vi "LoopselFF_2cam.VI"() -> ()   [LabVIEW 2017]
panel:
  in  "nob slide":u32(slide)=27666 scale=1.0..6.0
  in  "no.of blocks (nob)":u32=6
  out "cams recognised":u8
  in  "cam select\n1: cam 1\n2: cam 2\n3: both cams":u8=3
  out "Signalverlaufgraph 2":u16[](graph)=[0, 0, 0, 0, 0, 1, 0, 27665, 0, 0, 0, 0, 0, 0, 0, 0, 0, 0, 0, 0, 0, 0, 0, 0, 0, 0, 0, 0, 0, 0, 0, 0, 0, 0, 0, 0, 0, 0, 0, 0, 0, 0, 0, 0, 0, 0, 0, 0, 0, 0, 0, 0, 0, 0, 0, 0, 0, 0, 0, 0, 0, 0, 0, 0, 0, 0, 0, 0, 0, 0, 0, 0, 0, 0, 0, 0, 0, 0, 0, 0, 0, 0, 0, 0, 0, 0, 0, 0, 0, 0, 0, 0, 0, 0, 0, 0, 0, 0, 0, 0, 0, 0, 0, 0, 0, 0, 0, 0, 0, 0, 0, 0, 0, 0, 0, 0, 0, 0, 0, 0, 0, 0, 0, 0, 0, 0, 0, 0, 0, 0, 0, 0, 0, 0, 0, 0, 0, 0, 0, 0, 0, 0, 0, 0, 0, 0, 0, 0, 0, 0, 0, 0, 0, 0, 0, 0, 0, 0, 0, 0, 0, 0, 0, 0, 0, 0, 0, 0, 0, 0, 0, 0, 0, 0, 0, 0, 0, 0, 0, 0, 0, 0, 0, 0, 0, 0, 0, 0, 0, 0, 0, 0, 0, 0, 0, 0, 0, 0, 0, 0, 0, 0, 0, 0, 0, 0, 0, 0, 0, 0, 0, 0, 0, 0, 0, 0, 0, 0, 0, 0, 0, 0, 0, 0, 0, 0, 0, 0, 0, 0, 0, 0, 0, 0, 0, 0, 0, 0, 0, 0, 0, 0, 0, 0, 0, 0, 0, 0, 0, 0, 0, 0, 0, 0, 0, 0, 0, 0, 0, 0, 0, 0, 0, 0, 0, 0, 0, 0, 0, 0, 0, 0, 0, 0, 0, 0, 0, 0, 0, 0, 0, 0, 0, 0, 0, 0, 0, 0, 0, 0, 0, 0, 0, 0, 0, 0, 0, 0, 0, 0, 0, 0, 0, 0, 0, 0, 0, 0, 0, 0, 0, 0, 0, 0, 0, 0, 0, 0, 0, 0, 0, 0, 0, 0, 0, 0, 0, 0, 0, 0, 0, 0, 0, 0, 0, 0, 0, 0, 0, 0, 0, 0, 0, 0, 0, 0, 0, 0, 0, 0, 0, 0, 0, 0, 0, 0, 0, 0, 0, 0, 0, 0, 0, 0, 0, 0, 0, 0, 0, 0, 0, 0, 0, 0, 0, 0, 0, 0, 0, 0, 0, 0, 0, 0, 0, 0, 0, 0, 0, 0, 0, 0, 0, 0, 0, 0, 0, 0, 0, 0, 0, 0, 0, 0, 0, 0, 0, 0, 0, 0, 0, 0, 0, 0, 0, 0, 0, 0, 0, 0, 0, 0, 0, 0, 0, 0, 0, 0, 0, 0, 0, 0, 0, 0, 0, 0, 0, 0, 0, 0, 0, 0, 0, 0, 0, 0, 0, 0, 0, 0, 0, 0, 0, 0, 0, 0, 0, 0, 0, 0, 0, 0, 0, 0, 0, 0, 0, 0, 0, 0, 0, 0, 0, 0, 0, 0, 0, 0, 0, 0, 0, 0, 0, 0, 0, 0, 0, 0, 0, 0, 0, 0, 0, 0, 0, 0, 0, 0, 0, 0, 0, 0, 0, 0, 0, 0, 0, 0, 0, 0, 0, 0, 0, 0, 0, 0, 0, 0, 0, 0, 0, 0, 0, 0, 0, 0, 0, 0, 0, 0, 0, 0, 0, 0, 0, 0, 0, 0, 0, 0, 0, 0, 0, 0, 0, 0, 0, 0, 0, 0, 0, 0, 0, 0, 0, 0, 0, 0, 0, 0, 0, 0, 0, 0, 0, 0, 0, 0, 0, 0, 0, 0, 0, 0, 0, 0, 0, 0, 0, 0, 0, 0, 0, 0, 0, 0, 0, 0, 0, 0, 0, 0, 0, 0, 0, 0, 0, 0, 0, 0, 0, 0, 0, 0, 0, 0, 0, 0, 0, 0, 0, 0, 0, 0, 0, 0, 0, 0, 0, 0, 0, 0, 0, 0, 0, 0, 0, 0, 0, 0, 0, 0, 0, 0, 0, 0, 0, 0, 0, 0, 0, 0, 0, 0, 0, 0, 0, 0, 0, 0, 0, 0, 0, 0, 0, 0, 0, 0, 0, 0, 0, 0, 0, 0, 0, 0, 0, 0, 0, 0, 0, 0, 0, 0, 0, 0, 0, 0, 0, 0, 0, 0, 0, 0, 0, 0, 0, 0, 0, 0, 0, 0, 0, 0, 0, 0, 0, 0, 0, 0, 0, 0, 0, 0, 0, 0, 0, 0, 0, 0, 0, 0, 0, 0, 0, 0, 0, 0, 0, 0, 0, 0, 0, 0, 0, 0, 0, 0, 0, 0, 0, 0, 0, 0, 0, 0, 0, 0, 0, 0, 0, 0, 0, 0, 0, 0, 0, 0, 0, 0, 0, 0, 0, 0, 0, 0, 0, 0, 0, 0, 0, 0, 0, 0, 0, 0, 0, 0, 0, 0, 0, 0, 0, 0, 0, 0, 0, 0, 0, 0, 0, 0, 0, 0, 0, 0, 0, 0, 0, 0, 0, 0, 0, 0, 0, 0, 0, 0, 0, 0, 0, 0, 0, 0, 0, 0, 0, 0, 0, 0, 0, 0, 0, 0, 0, 0, 0, 0, 0, 0, 0, 0, 0, 0, 0, 0, 0, 0, 0, 0, 0, 0, 0, 0, 0, 0, 0, 0, 0, 0, 0, 0, 0, 0, 0, 0, 0, 0, 0, 0, 0, 0, 0, 0, 0, 0, 0, 0, 0, 0, 0, 0, 0, 0, 0, 0, 0, 0, 0, 0, 0, 0, 0, 0, 0, 0, 0, 0, 0, 0, 0, 0, 0, 0, 0, 0, 0, 0, 0, 0, 0, 0, 0, 0, 0, 0, 0, 0, 0, 0, 0, 0, 0, 0, 0, 0, 0, 0, 0, 0, 0, 0, 0, 0, 0, 0, 0, 0, 0, 0, 0, 0, 0, 0, 0, 0, 0, 0, 0, 0, 0, 0, 0, 0, 0, 0, 0, 0, 0, 0, 0, 0, 0, 0, 0, 0, 0, 0, 0, 0, 0, 0, 0, 0, 0, 0, 0, 0, 0, 0, 0, 0, 0, 0, 0, 0, 0, 0, 0, 0, 0, 0, 0, 0, 0, 0, 0, 0, 0, 0, 0, 0, 0, 0, 0, 0, 0, 0, 0, 0, 0, 0, 0, 0, 0, 0, 0, 0, 0, 0, 0, 0, 0, 0, 0, 0, 0, 0, 0, 0, 0, 0, 0, 0, 0, 0, 0, 0, 0, 0, 0, 0, 0, 0, 0, 0, 0, 0, 0, 0, 0, 0, 0, 0, 0, 0, 0, 0, 0, 0, 0, 0, 0, 0, 0, 0, 0, 0, 0, 0, 0, 0, 0, 0, 0, 0, 0, 0, 0, 0, 0, 0, 0, 0, 0, 0, 0, 0, 0, 0, 0, 0, 0, 0, 0, 0, 0, 0, 0, 0, 0, 0, 0, 0, 0, 0, 0, 0]
  in  "alloc mem":bool
  out "FREE \nRAM MB":u64=14179
  out "BUILT-IN\nRAM MB":u64=16662
  out "SEC":dbl=1.2
  out "MB RAM":u64=125
  in  "pos slope":u8=1
  in  "both slopes":u8
  in  "DAT in 10ns":u32
  in  "extTrig 0/1":u8
  in  "stop all":bool
  in  "start new block":bool
  in  "nos slide":u32(slide)=27666 scale=1.0..70000.0
  in  "frequency[Hz]":u32
  in  "no.of samples (nos)":u32=10000
  in  "exposuretime[ms]":dbl=0.02 format="%.3f"
  out "Signalverlaufgraph":u16[](graph)=[0, 0, 0, 0, 0, 1, 0, 27665, 0, 0, 0, 0, 0, 0, 0, 0, 0, 0, 0, 0, 0, 0, 0, 0, 0, 0, 0, 0, 0, 0, 0, 0, 0, 0, 0, 0, 0, 0, 0, 0, 0, 0, 0, 0, 0, 0, 0, 0, 0, 0, 0, 0, 0, 0, 0, 0, 0, 0, 0, 0, 0, 0, 0, 0, 0, 0, 0, 0, 0, 0, 0, 0, 0, 0, 0, 0, 0, 0, 0, 0, 0, 0, 0, 0, 0, 0, 0, 0, 0, 0, 0, 0, 0, 0, 0, 0, 0, 0, 0, 0, 0, 0, 0, 0, 0, 0, 0, 0, 0, 0, 0, 0, 0, 0, 0, 0, 0, 0, 0, 0, 0, 0, 0, 0, 0, 0, 0, 0, 0, 0, 0, 0, 0, 0, 0, 0, 0, 0, 0, 0, 0, 0, 0, 0, 0, 0, 0, 0, 0, 0, 0, 0, 0, 0, 0, 0, 0, 0, 0, 0, 0, 0, 0, 0, 0, 0, 0, 0, 0, 0, 0, 0, 0, 0, 0, 0, 0, 0, 0, 0, 0, 0, 0, 0, 0, 0, 0, 0, 0, 0, 0, 0, 0, 0, 0, 0, 0, 0, 0, 0, 0, 0, 0, 0, 0, 0, 0, 0, 0, 0, 0, 0, 0, 0, 0, 0, 0, 0, 0, 0, 0, 0, 0, 0, 0, 0, 0, 0, 0, 0, 0, 0, 0, 0, 0, 0, 0, 0, 0, 0, 0, 0, 0, 0, 0, 0, 0, 0, 0, 0, 0, 0, 0, 0, 0, 0, 0, 0, 0, 0, 0, 0, 0, 0, 0, 0, 0, 0, 0, 0, 0, 0, 0, 0, 0, 0, 0, 0, 0, 0, 0, 0, 0, 0, 0, 0, 0, 0, 0, 0, 0, 0, 0, 0, 0, 0, 0, 0, 0, 0, 0, 0, 0, 0, 0, 0, 0, 0, 0, 0, 0, 0, 0, 0, 0, 0, 0, 0, 0, 0, 0, 0, 0, 0, 0, 0, 0, 0, 0, 0, 0, 0, 0, 0, 0, 0, 0, 0, 0, 0, 0, 0, 0, 0, 0, 0, 0, 0, 0, 0, 0, 0, 0, 0, 0, 0, 0, 0, 0, 0, 0, 0, 0, 0, 0, 0, 0, 0, 0, 0, 0, 0, 0, 0, 0, 0, 0, 0, 0, 0, 0, 0, 0, 0, 0, 0, 0, 0, 0, 0, 0, 0, 0, 0, 0, 0, 0, 0, 0, 0, 0, 0, 0, 0, 0, 0, 0, 0, 0, 0, 0, 0, 0, 0, 0, 0, 0, 0, 0, 0, 0, 0, 0, 0, 0, 0, 0, 0, 0, 0, 0, 0, 0, 0, 0, 0, 0, 0, 0, 0, 0, 0, 0, 0, 0, 0, 0, 0, 0, 0, 0, 0, 0, 0, 0, 0, 0, 0, 0, 0, 0, 0, 0, 0, 0, 0, 0, 0, 0, 0, 0, 0, 0, 0, 0, 0, 0, 0, 0, 0, 0, 0, 0, 0, 0, 0, 0, 0, 0, 0, 0, 0, 0, 0, 0, 0, 0, 0, 0, 0, 0, 0, 0, 0, 0, 0, 0, 0, 0, 0, 0, 0, 0, 0, 0, 0, 0, 0, 0, 0, 0, 0, 0, 0, 0, 0, 0, 0, 0, 0, 0, 0, 0, 0, 0, 0, 0, 0, 0, 0, 0, 0, 0, 0, 0, 0, 0, 0, 0, 0, 0, 0, 0, 0, 0, 0, 0, 0, 0, 0, 0, 0, 0, 0, 0, 0, 0, 0, 0, 0, 0, 0, 0, 0, 0, 0, 0, 0, 0, 0, 0, 0, 0, 0, 0, 0, 0, 0, 0, 0, 0, 0, 0, 0, 0, 0, 0, 0, 0, 0, 0, 0, 0, 0, 0, 0, 0, 0, 0, 0, 0, 0, 0, 0, 0, 0, 0, 0, 0, 0, 0, 0, 0, 0, 0, 0, 0, 0, 0, 0, 0, 0, 0, 0, 0, 0, 0, 0, 0, 0, 0, 0, 0, 0, 0, 0, 0, 0, 0, 0, 0, 0, 0, 0, 0, 0, 0, 0, 0, 0, 0, 0, 0, 0, 0, 0, 0, 0, 0, 0, 0, 0, 0, 0, 0, 0, 0, 0, 0, 0, 0, 0, 0, 0, 0, 0, 0, 0, 0, 0, 0, 0, 0, 0, 0, 0, 0, 0, 0, 0, 0, 0, 0, 0, 0, 0, 0, 0, 0, 0, 0, 0, 0, 0, 0, 0, 0, 0, 0, 0, 0, 0, 0, 0, 0, 0, 0, 0, 0, 0, 0, 0, 0, 0, 0, 0, 0, 0, 0, 0, 0, 0, 0, 0, 0, 0, 0, 0, 0, 0, 0, 0, 0, 0, 0, 0, 0, 0, 0, 0, 0, 0, 0, 0, 0, 0, 0, 0, 0, 0, 0, 0, 0, 0, 0, 0, 0, 0, 0, 0, 0, 0, 0, 0, 0, 0, 0, 0, 0, 0, 0, 0, 0, 0, 0, 0, 0, 0, 0, 0, 0, 0, 0, 0, 0, 0, 0, 0, 0, 0, 0, 0, 0, 0, 0, 0, 0, 0, 0, 0, 0, 0, 0, 0, 0, 0, 0, 0, 0, 0, 0, 0, 0, 0, 0, 0, 0, 0, 0, 0, 0, 0, 0, 0, 0, 0, 0, 0, 0, 0, 0, 0, 0, 0, 0, 0, 0, 0, 0, 0, 0, 0, 0, 0, 0, 0, 0, 0, 0, 0, 0, 0, 0, 0, 0, 0, 0, 0, 0, 0, 0, 0, 0, 0, 0, 0, 0, 0, 0, 0, 0, 0, 0, 0, 0, 0, 0, 0, 0, 0, 0, 0, 0, 0, 0, 0, 0, 0, 0, 0, 0, 0, 0, 0, 0, 0, 0, 0, 0, 0, 0, 0, 0, 0, 0, 0, 0, 0, 0, 0, 0, 0, 0, 0, 0, 0, 0, 0, 0, 0, 0, 0, 0, 0, 0, 0, 0, 0, 0, 0, 0, 0, 0, 0, 0, 0, 0, 0, 0, 0, 0, 0, 0, 0, 0, 0, 0, 0, 0, 0, 0, 0, 0, 0, 0, 0, 0, 0, 0, 0, 0, 0, 0, 0, 0, 0, 0, 0, 0, 0, 0, 0, 0, 0, 0, 0, 0, 0, 0, 0, 0, 0, 0, 0, 0, 0, 0, 0, 0, 0, 0, 0, 0, 0, 0, 0, 0, 0, 0, 0, 0, 0, 0, 0, 0, 0, 0, 0, 0, 0, 0, 0, 0, 0, 0, 0, 0, 0, 0, 0, 0, 0, 0, 0, 0, 0, 0, 0, 0, 0, 0, 0, 0, 0, 0, 0, 0, 0, 0, 0, 0, 0, 0, 0, 0, 0, 0, 0, 0, 0, 0, 0, 0, 0, 0, 0, 0, 0, 0, 0, 0, 0, 0, 0, 0, 0, 0, 0]
  # "Start with run"
  # "Abort with ESC"
  # "press Esc to stop measurement"
  # "1x"
  # "exit here"
  # "repeat"
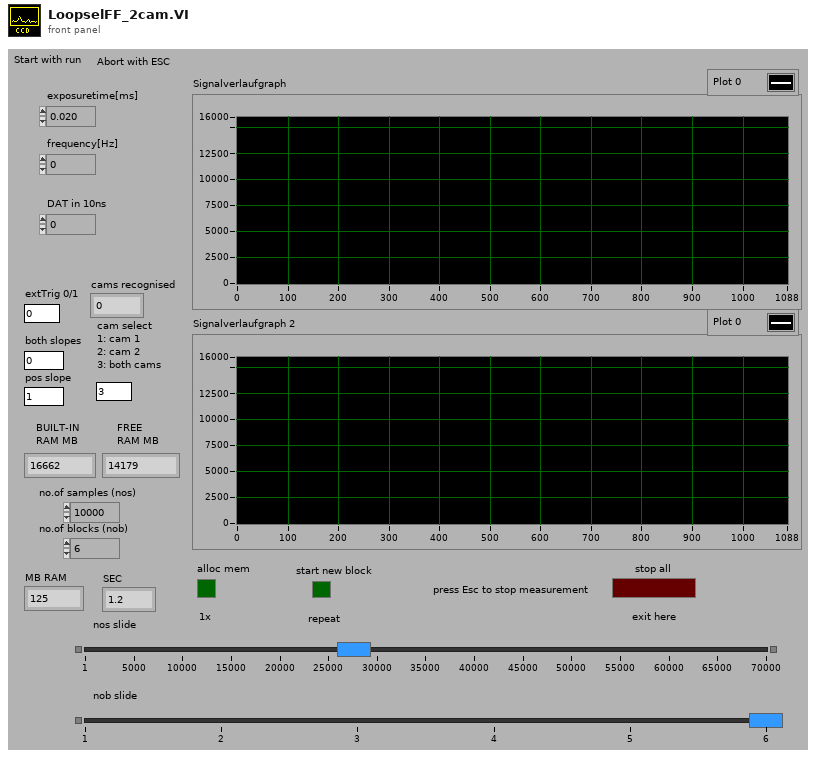
[diagram p1: front panel]
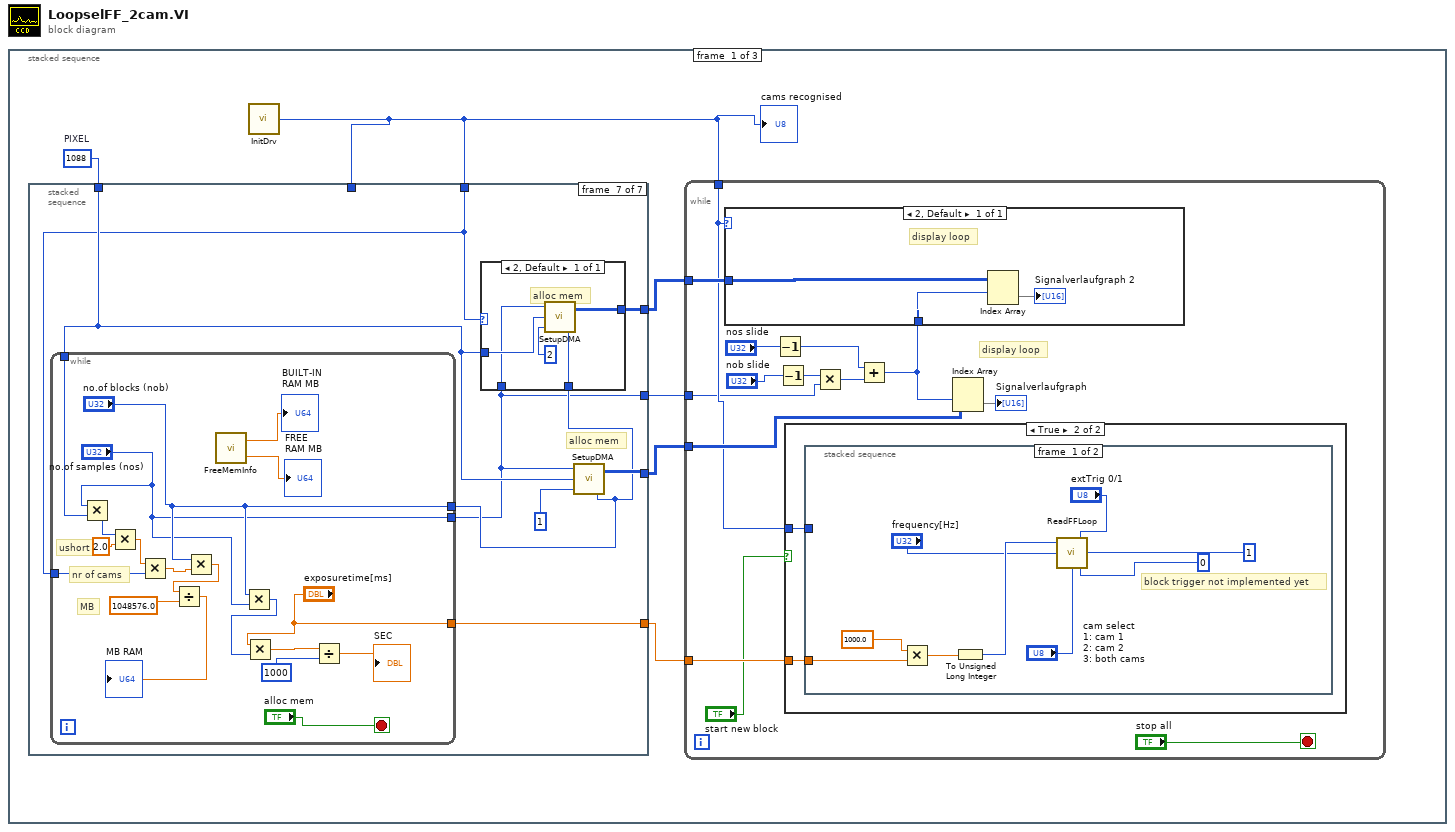
[diagram p0: block diagram]
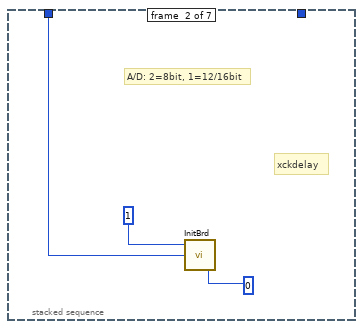
[diagram p5: hidden frame]
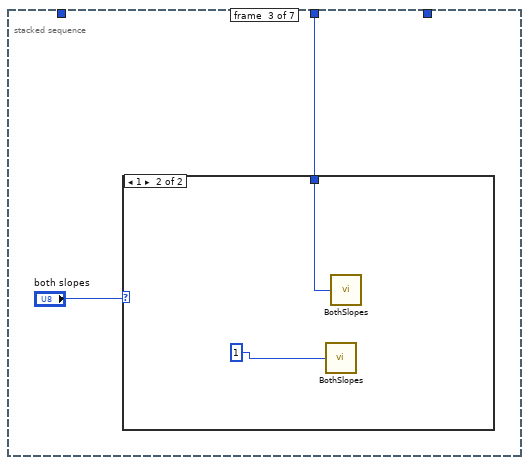
[diagram p6: hidden frame]
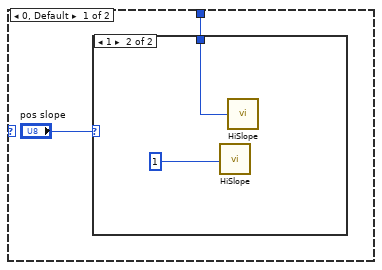
[diagram p7: hidden frame]
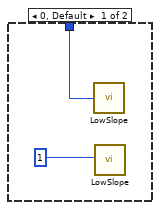
[diagram p8: hidden frame]
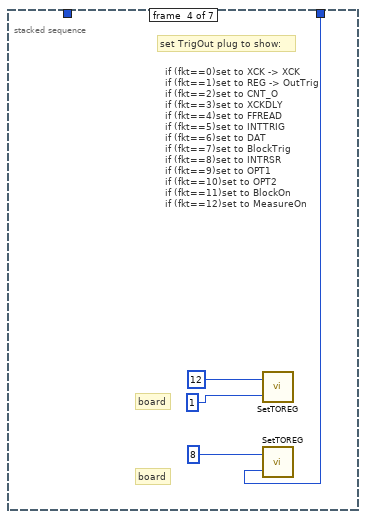
[diagram p9: hidden frame]
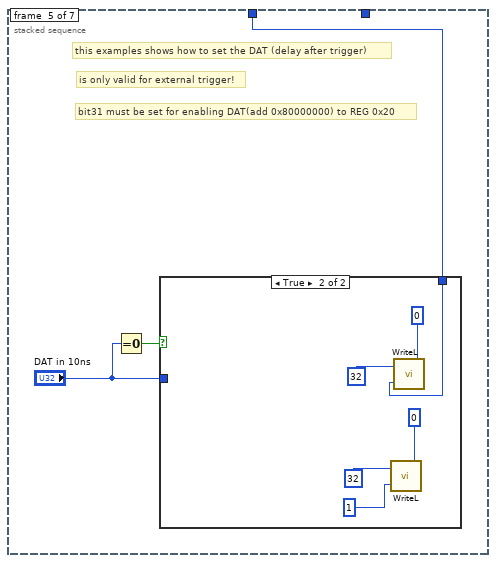
[diagram p10: hidden frame]
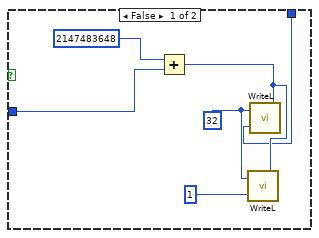
[diagram p11: hidden frame]
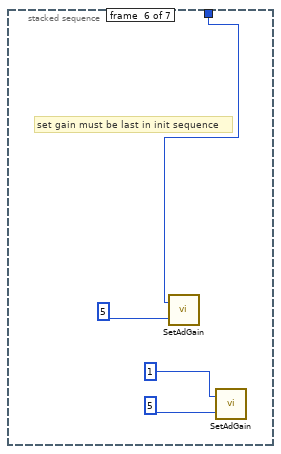
[diagram p12: hidden frame]
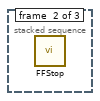
[diagram p13: hidden frame]
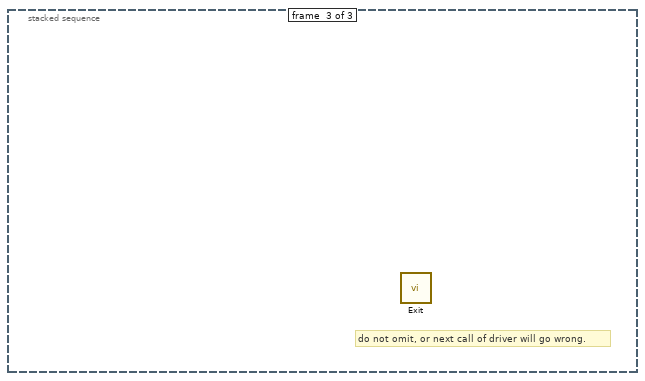
[diagram p14: hidden frame]
diagram:
  n1 = stacked-sequence {
    frame #0 {
      w6 = u32 1088  # PIXEL
      n2 = call "InitDrv.vi"() -> ("Boards"=w2:u8)  [unwired: 1 in]
      "cams recognised" <- w2
      n3 = stacked-sequence {
        tunnel: [_ _ _ _ _ _ w78] -> w3
        tunnel: w6 -> [_ w35 _ _ _ _ w76]
        tunnel: w2 -> [_ _ _ _ _ _ w73]
        tunnel: [_ _ _ _ _ _ w75] -> w5
        tunnel: [_ _ _ _ _ _ w74] -> w4
        tunnel: w2 -> [_ _ w38 w48 w52 w67 _]
        tunnel: [_ _ _ _ _ _ w71] -> w1
        frame #0 {
        }
        frame #1 {
          # "xckdelay"
          # "A/D: 2=8bit, 1=12/16bit"
          n4 = call "InitBrd.vi"("xckdly"=u32 0, "pixel"=w35, "flag816"=u32 1) -> ()  [unwired: 3 in]
        }
        frame #2 {
          n5 = case shown="1" "both slopes" {
            tunnel: w38 -> [w40 w47]
            frame 0, Default {
              n6 = case shown="1" "pos slope" {
                tunnel: w40 -> [w43 w45]
                frame 0, Default {
                  n7 = call "LowSlope.vi"("board"=w43) -> ()  [unwired: 1 in]
                  n8 = call "LowSlope.vi"("board"=1) -> ()  [unwired: 1 in]
                }
                frame 1 {
                  n9 = call "HiSlope.vi"("board"=1) -> ()  [unwired: 1 in]
                  n10 = call "HiSlope.vi"("board"=w45) -> ()  [unwired: 1 in]
                }
              }
            }
            frame 1 {
              n11 = call "BothSlopes.vi"("board"=1) -> ()  [unwired: 1 in]
              n12 = call "BothSlopes.vi"("board"=w47) -> ()  [unwired: 1 in]
            }
          }
        }
        frame #3 {
          # "board"
          # "board"
          # "set TrigOut plug to show:"
          # "if (fkt==0)set to XCK -> XCK\nif (fkt==1)set to REG -> OutTrig\nif (fkt==2)set to CNT_O\nif (fkt==3)set to XCKDLY\nif (fkt==4)set to FFREAD\nif (fkt==5)set to INTTRIG\nif (fkt==6)set to DAT\nif (fkt==7)set to BlockTrig\nif (fkt==8)set to INTRSR\nif (fkt==9)set to OPT1\nif (fkt==10)set to OPT2\nif (fkt==11)set to BlockOn\nif (fkt==12)set to MeasureOn"
          n13 = call "SetTOREG.vi"("board"=u8 1, "fkt"=u8 12) -> ()  [unwired: 1 in]
          n14 = call "SetTOREG.vi"("board"=w48, "fkt"=u8 8) -> ()  [unwired: 1 in]
        }
        frame #4 {
          # "bit31 must be set for enabling DAT(add 0x80000000) to REG 0x20"
          # "is only valid for external trigger!"
          # "this examples shows how to set the DAT (delay after trigger)"
          n15 = Equal To 0?(x="DAT in 10ns") -> (x = 0?=w54:bool)
          n16 = case shown="True" w54 {
            tunnel: "DAT in 10ns" -> [w59 _]
            tunnel: w52 -> [w56 w64]
            frame False {
              w58 = u32 32
              n17 = Add(x=u32 2147483648, y=w59) -> (x+y=w57:u32)
              n18 = call "WriteL.vi"("val"=w57, "board"=1, "offset"=w58) -> ()
              n19 = call "WriteL.vi"("val"=w57, "board"=w56, "offset"=w58) -> ()
            }
            frame True {
              n20 = call "WriteL.vi"("val"=0, "board"=1, "offset"=u32 32) -> ()
              n21 = call "WriteL.vi"("val"=0, "board"=w64, "offset"=u32 32) -> ()
            }
          }
        }
        frame #5 {
          # "set gain must be last in init sequence"
          n22 = call "SetAdGain.vi"("gain"=u8 5, "board"=w67) -> ()  [unwired: 1 in]
          n23 = call "SetAdGain.vi"("gain"=u8 5, "board"=u8 1) -> ()  [unwired: 1 in]
        }
        frame #6 {
          # "alloc mem"
          n24 = while {
            tunnel: w76 -> [w99]
            tunnel: ["exposuretime[ms]"] -> w78
            tunnel: ["no.of samples (nos)"] -> w71
            tunnel: w73 -> [w89]
            tunnel: ["no.of blocks (nob)"] -> w72
            stop <- "alloc mem" stop-if-true
            # "MB"
            # "nr of cams"
            # "ushort"
            n25 = Multiply(x="no.of samples (nos)", y=w99) -> (x*y=w100:u32)
            n26 = Multiply(x=w100, y=2.0) -> (x*y=w90:dbl)
            n27 = Multiply(x=w90, y=w89) -> (x*y=w88:dbl)
            n28 = Multiply(x="no.of blocks (nob)", y=w88) -> (x*y=w87:dbl)
            n29 = Divide(x=w87, y=1048576.0) -> (x/y=→"MB RAM":dbl)
            n30 = call "FreeMemInfo.vi"() -> ("PhysicalSpace"=→"BUILT-IN\nRAM MB":dbl, "PhysicalFreeSpace"=→"FREE \nRAM MB":dbl)  [unwired: 1 in]
            n31 = Multiply(x="no.of blocks (nob)", y="no.of samples (nos)") -> (x*y=w84:u32)
            n32 = Multiply(x="exposuretime[ms]", y=w84) -> (x*y=w96:dbl)
            n33 = Divide(x=w96, y=1000) -> (x/y=→"SEC":dbl)
          }
          n34 = case shown="2, Default" w73 {
            tunnel: w76 -> [w82]
            tunnel: w71 -> [w81]
            tunnel: [w80] -> w75
            tunnel: w72 -> [w79]
            frame 2, Default {
              # "alloc mem"
              n35 = call "SetupDMA.vi"("blocks"=w79, "Drv"=u32 2, "pixel"=w82, "nos"=w81) -> ("Data Values"=w80:u16[][])
            }
          }
          n36 = call "SetupDMA.vi"("blocks"=w72, "Drv"=u32 1, "pixel"=w76, "nos"=w71) -> ("Data Values"=w74:u16[][])
        }
      }
      n37 = while {
        tunnel: w5 -> [w18]
        tunnel: w4 -> [w17]
        tunnel: w3 -> [w15]
        tunnel: w2 -> [w14]
        tunnel: w1 -> [w10]
        stop <- "stop all" stop-if-true
        # "display loop"
        n38 = Decrement(x="nos slide") -> (x-1=w8:u32)
        n39 = Decrement(x="nob slide") -> (x-1=w11:u32)
        n40 = case shown="True" "start new block" {
          tunnel: w15 -> [_ w22]
          tunnel: w14 -> [_ w21]
          frame False {
          }
          frame True {
            n41 = stacked-sequence {
              tunnel: w22 -> [w24 _]
              tunnel: w21 -> [_ _]
              frame #0 {
                # "block trigger not implemented yet"
                n42 = Multiply(x=1000.0, y=w24) -> (x*y=w26:dbl)
                n43 = To Unsigned Long Integer(number=w26) -> (unsigned 32bit integer=w31:u32)
                n44 = call "ReadFFLoop.vi"("blocktrigger"=u8 0, "btrig_ch"=u8 1, "ExtTrig"="extTrig 0/1", "cam_sel"="cam select\n1: cam 1\n2: cam 2\n3: both cams", "freq"="frequency[Hz]", "exptus"=w31) -> ()
              }
              frame #1 {
              }
            }
          }
        }
        n45 = Multiply(x=w11, y=w10) -> (x*y=w9:u32)
        n46 = Add(x=w8, y=w9) -> (x+y=w7:u32)
        n47 = case shown="2, Default" w14 {
          tunnel: w7 -> [w34]
          tunnel: w18 -> [w33]
          frame 2, Default {
            # "display loop"
            n48 = Index Array(array=w33, index (row)=w34) -> (element=→"Signalverlaufgraph 2":u16[])  [unwired: 1 in]
          }
        }
        n49 = Index Array(array=w17, index (row)=w7) -> (element=→"Signalverlaufgraph":u16[])  [unwired: 1 in]
      }
    }
    frame #1 {
      n50 = call "FFStop.vi"() -> ()  [unwired: 1 in]
    }
    frame #2 {
      # "do not omit, or next call of driver will go wrong."
      n51 = call "Exit.vi"() -> ()  [unwired: 1 in]
    }
  }
